vi "Set To.vi"(8 "error in (no error)":errorcluster, 10 "To":T1[](array[typedef]), 11 "Gmail in":refnum<class "Gmail.lvclass">) -> (0 "error out":errorcluster, 3 "Gmail out":refnum<class "Gmail.lvclass">)   [LabVIEW 2020, in "Gmail API.lvlib" / "Gmail.lvclass"]
uses:
  Gmail.lvclass
  Mail Address.ctl
  Gmail.lvclass/Gmail.ctl
  Gmail API.lvlib
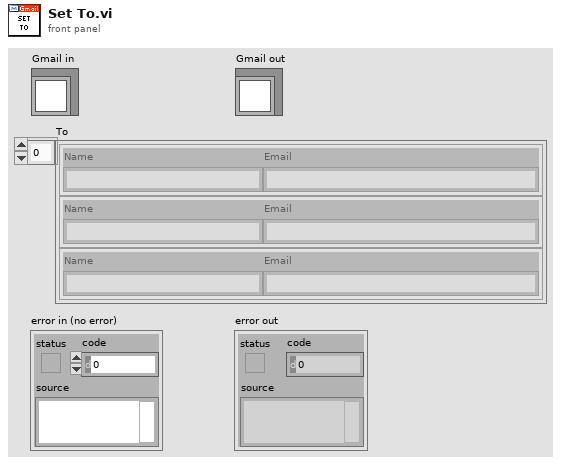
[diagram p1: front panel]
types:
  T1 = typedef "Gmail API.lvlib/Mail Address.ctl" = cluster{"Name":string, "Email":string}
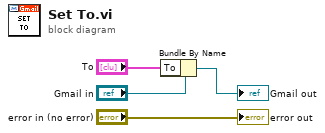
[diagram p0: block diagram]
diagram:
  n1 = Bundle By Name(cluster="Gmail in", "To"="To") -> (→"Gmail out":refnum<class "Gmail.lvclass">)
  "error out" <- "error in (no error)"
